vi "getDescription.vi"(8 "error in (no error)":errorcluster, 11 "Decaf in":refnum<class "Decaf.lvclass">) -> (0 "error out":errorcluster, 2 "description":string="Decaf", 3 "Decaf out":refnum<class "Decaf.lvclass">)   [LabVIEW 2018, in "Decaf.lvclass"]
uses:
  Decaf.lvclass
  Beverage Class/Beverage.lvclass
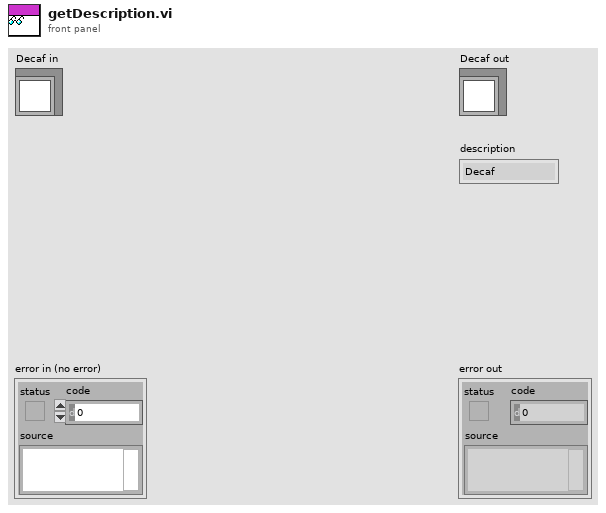
[diagram p1: front panel]
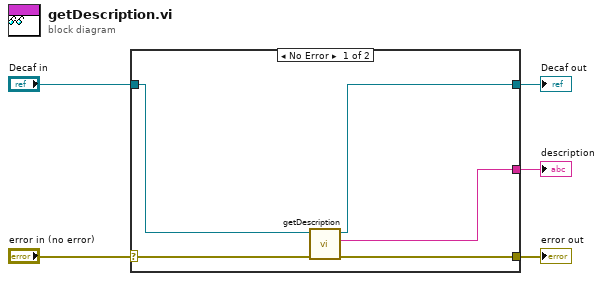
[diagram p0: block diagram]
diagram:
  n1 = case shown="No Error" "error in (no error)" {
    selector: "error in (no error)" -> [w10 w11]
    tunnel: [w9 w11] -> w4
    tunnel: [w7 w12] -> w2
    tunnel: "Decaf in" -> [w8 w12]
    tunnel: [w6 _] -> w1
    frame No Error {
      n2 = call-parent "getDescription.vi"("error in (no error)"=w10, "Beverage in"=w8) -> ("error out"=w9:errorcluster, "description"=w6:string, "Beverage out"=w7:refnum<class "Decaf.lvclass">)  [unwired: 7 in]
    }
    frame Error {
    }
  }
  "error out" <- w4
  "Decaf out" <- w2
  "description" <- w1
